vi "Get All CD Parameters.vi"(8 "error in (no error)":errorcluster, 11 "Device Reference in":T17 format="%.0x") -> (0 "error out":errorcluster, 2 "VS References":T1={"Properties"={"Name"="", "CAN"={"Database File"=path "", "CAN Interface"=enum."CAN1", "Baud Rate"=0, "Diagnostic Protocol"=enum."GMLAN", "Transport Protocol"=enum."ISO TP - Normal Mode", "Transmit ID"=0, "Receive ID"=0, "Transmit Extension"=2, "Receive Extension"=1, "Receive UUDT ID"=0, "Enable Stream"=TRUE, "VW TP Channel ID"=0, "Security"={"DLL Path"=path "", "Security Level"=0}}, "FPGA Settings"={"RT Bitfile Path"=path "", "RIO Device"=0, "Enable"=FALSE}, "PIDs"=[], "PID Lookup"=variant(enum16{"GMLAN", "KWP-2000", "UDS"} enum."GMLAN"), "CPIDs"=[], "CPID Lookup"=variant(u32 0), "DIDs"=[], "DID Lookup"=variant(u8 0), "DPIDs"=[], "DPID Lookup"=variant(u32 0), "DTC descriptor"={"DTC Byte Length"=2, "Status Byte Length"=1, "Add Data Byte Length"=1, "Byte Order"=enum."Motorola"}}, "Refs"={"PIDs"=[], "CPIDs"={"Refs"=[], "Values"=[]}, "DIDs"=[], "Number of DTCs"=0, "DTCs"=[], "Success"=0, "Command Chanels"=[]}} {"Refs"."Command Chanels" format="%.0x"; "Refs"."Success" format="%.0x"; "Refs"."DTCs" format="%.0x"; "Refs"."Number of DTCs" format="%.0x"; "Refs"."DIDs" format="%.0x"; "Refs"."CPIDs"."Refs"."Data Reference" format="%.0x"; "Refs"."PIDs" format="%.0x"; "Properties"."CPIDs"."Signals"."Byte Order" items=["Little Endian", "Big Endian"]; "Properties"."CPIDs"."Signals"."Data Type" items=["Signed", "Unsigned", "IEEE Float"]; "Properties"."DIDs"."Signals"."Byte Order" items=["Little Endian", "Big Endian"]; "Properties"."DIDs"."Signals"."Data Type" items=["Signed", "Unsigned", "IEEE Float"]; "Properties"."CAN"."VW TP Channel ID" format="%.0x"; "Properties"."CAN"."Receive UUDT ID" format="%.0x"; "Properties"."CAN"."Receive Extension" format="%.0x"; "Properties"."CAN"."Transmit Extension" format="%.0x"; "Properties"."CAN"."Receive ID" format="%.0x"; "Properties"."CAN"."Transmit ID" format="%.0x"; "Properties"."PIDs"."Signals"."Byte Order" items=["Little Endian", "Big Endian"]; "Properties"."PIDs"."Signals"."Data Type" items=["Signed", "Unsigned", "IEEE Float"]}, 3 "Device Reference out":T17 format="%.0x")   [LabVIEW 2015, in "Diagnostics Addon System Explorer.lvlib"]
uses:
  System Explorer/Diagnostics Addon System Explorer.lvlib
  <vilib>/NI Veristand/Custom Device API/Custom Device Item Ref.ctl
  Compiled.Settings
  Section Properties.ctl
  Shared/CAN Configuration.ctl
  Shared/CAN Interface.ctl
  Shared/Diagnostic Protocols.ctl
  Shared/Transport Protocols.ctl
  Shared/Security.ctl
  Shared/FPGA Bitfile Settings.ctl
  Shared/Frame Parameters.ctl
  Shared/Signal Parameters.ctl
  Shared/DPID Parameters.ctl
  Shared/DPID Periodic Rate.ctl
  <vilib>/Automotive Diagnostic Command Set/Diagnostic Protocols.llb/DTC Descriptor.ctl
  Shared/Compiled.Refs.ctl
  <vilib>/NI Veristand/Custom Device API/Data Reference.ctl
  <vilib>/NI Veristand/Custom Device API/Block Data Reference.ctl
  <vilib>/NI Veristand/Custom Device API/Data Access Type.ctl
  Shared/FG Action.ctl
  Shared/ID FG.vi
  Shared/Get Frame.vi
  System Explorer/SubVIs/Calculate Frame Size.vi
  Shared/Get Signals.vi
  Shared/Signal Parameters FG.vi
  <vilib>/NI Veristand/Custom Device API/NI VeriStand - Get Item Property.vi
  <vilib>/NI Veristand/Custom Device API/Get Item Property (U32 Array).vi
  <vilib>/NI Veristand/Custom Device API/Get Item Property (U32).vi
  <vilib>/NI Veristand/Custom Device API/NI VeriStand - Set Item Property.vi
  <vilib>/NI Veristand/Custom Device API/Set Item Property (U32).vi
  Shared/GUID Lookup.vi
  <vilib>/NI Veristand/Custom Device API/Set Item Property (U32 Array).vi
  <vilib>/NI Veristand/Custom Device Tools/Custom Device Utility Library/NI VeriStand - Search for Item by GUID.vi
  <vilib>/NI Veristand/Custom Device API/Set Item Property (Path).vi
  <vilib>/NI Veristand/Custom Device API/Set Item Property (Boolean).vi
  <vilib>/NI Veristand/Custom Device API/Get Item Property (Path).vi
  <vilib>/NI Veristand/Custom Device API/Get Item Property (Boolean).vi
  <vilib>/NI Veristand/Custom Device Tools/Custom Device Utility Library/NI VeriStand - Search for Item by Name.vi
  <vilib>/NI Veristand/Custom Device API/Get Item Property (I32).vi
  <vilib>/NI Veristand/Custom Device API/Set Item Property (I32).vi
  <vilib>/NI Veristand/Custom Device API/NI VeriStand - Get Custom Device Channel Data.vi
  <vilib>/NI Veristand/Custom Device API/NI VeriStand - Get Item Description.vi
  <vilib>/NI Veristand/Custom Device API/Get Item Property (String).vi
  <vilib>/NI Veristand/Custom Device API/Get Item Property (Double).vi
  <vilib>/NI Veristand/Custom Device API/Set Item Property (String).vi
  <vilib>/NI Veristand/Custom Device API/Set Item Property (Double).vi
  <vilib>/NI Veristand/Custom Device API/NI VeriStand - Get Channel Block Data References.vi
  <vilib>/NI Veristand/Custom Device Tools/Custom Device Utility Library/Custom Device Utility Library.lvlib
  Shared/Diagnostics Addon Shared.lvlib
  <vilib>/NI Veristand/Custom Device API/Custom Device API.lvlib
  Diagnostics Addon Engine.lvlib
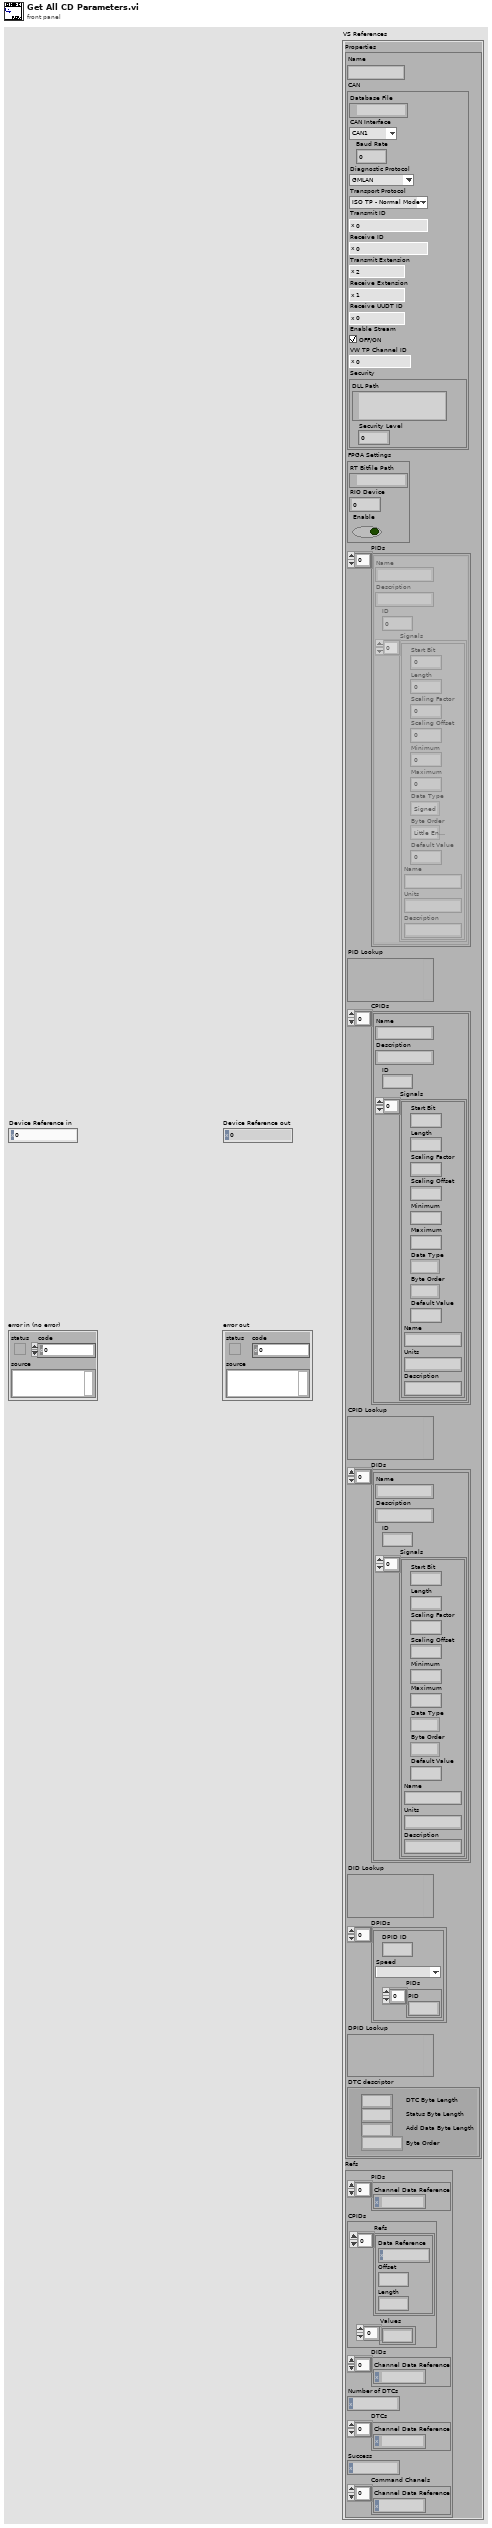
[diagram p1: front panel]
types:
  T1 = typedef "Diagnostics Addon Shared.lvlib/Compiled.Settings" = cluster{"Properties":T2, "Refs":T14}
  T2 = typedef "Diagnostics Addon Engine.lvlib/Section Properties.ctl" = cluster{"Name":string, "CAN":T3, "FPGA Settings":T8, "PIDs":T9[], "PID Lookup":variant, "CPIDs":T9[], "CPID Lookup":variant, "DIDs":T9[], "DID Lookup":variant, "DPIDs":T11[], "DPID Lookup":variant, "DTC descriptor":T13}
  T3 = typedef "Diagnostics Addon Shared.lvlib/CAN Configuration.ctl" = cluster{"Database File":path, "CAN Interface":T4, "Baud Rate":u32, "Diagnostic Protocol":T5, "Transport Protocol":T6, "Transmit ID":u32, "Receive ID":u32, "Transmit Extension":u8, "Receive Extension":u8, "Receive UUDT ID":u32, "Enable Stream":bool, "VW TP Channel ID":u32, "Security":T7}
  T4 = typedef "Diagnostics Addon Shared.lvlib/CAN Interface.ctl" = enum16{"CAN0", "CAN1", "CAN2", "CAN3", "CAN4", "CAN5", "CAN6", "CAN7", "CAN8", "CAN9", "CAN10", "CAN11", "CAN12", "CAN13", "CAN14", "CAN15", "CAN16", "CAN17", "CAN18", "CAN19", "CAN20", "CAN21", "CAN22", "CAN23", "CAN24", "CAN25", "CAN26", "CAN27", "CAN28", "CAN29", "CAN30", "CAN31", "CAN32", "CAN33", "CAN34", "CAN35", "CAN36", "CAN37", "CAN38", "CAN39", "CAN40", "CAN41", "CAN42", "CAN43", "CAN44", "CAN45", "CAN46", "CAN47", "CAN48", "CAN49", "CAN50", "CAN51", "CAN52", "CAN53", "CAN54", "CAN55", "CAN56", "CAN57", "CAN58", "CAN59", "CAN60", "CAN61", "CAN62", "CAN63", "CAN 256 (Virtual)", "CAN 257 (Virtual)"}
  T5 = typedef "Diagnostics Addon Shared.lvlib/Diagnostic Protocols.ctl" = enum16{"GMLAN", "KWP-2000", "UDS"}
  T6 = typedef "Diagnostics Addon Shared.lvlib/Transport Protocols.ctl" = enum16{"ISO TP - Normal Mode", "ISO TP - Mixed Mode", "VW TP 2.0", "Diagnostics on IP"}
  T7 = typedef "Diagnostics Addon Shared.lvlib/Security.ctl" = cluster{"DLL Path":path, "Security Level":u8}
  T8 = typedef "Diagnostics Addon Shared.lvlib/FPGA Bitfile Settings.ctl" = cluster{"RT Bitfile Path":path, "RIO Device":u16, "Enable":bool}
  T9 = typedef "Diagnostics Addon Shared.lvlib/Frame Parameters.ctl" = cluster{"Name":string, "Description":string, "ID":u16, "Signals":T10[]}
  T10 = typedef "Diagnostics Addon Shared.lvlib/Signal Parameters.ctl" = cluster{"Start Bit":u8, "Length":u8, "Scaling Factor":dbl, "Scaling Offset":dbl, "Minimum":dbl, "Maximum":dbl, "Data Type":u32, "Byte Order":u32, "Default Value":dbl, "Name":string, "Units":string, "Description":string}
  T11 = typedef "Diagnostics Addon Shared.lvlib/DPID Parameters.ctl" = cluster{"DPID ID":u8, "Speed":T12, "PIDs":u16[]}
  T12 = typedef "Diagnostics Addon Shared.lvlib/DPID Periodic Rate.ctl" = enum16{"Slow", "Medium", "Fast"}
  T13 = typedef "Diagnostics Addon Shared.lvlib/DTC Descriptor.ctl" = cluster{"DTC Byte Length":i32, "Status Byte Length":i32, "Add Data Byte Length":i32, "Byte Order":enum16{"Motorola", "Intel"}}
  T14 = typedef "Diagnostics Addon Shared.lvlib/Compiled.Refs.ctl" = cluster{"PIDs":T15[], "CPIDs":cluster{"Refs":T16[], "Values":dbl[]}, "DIDs":T15[], "Number of DTCs":T15, "DTCs":T15[], "Success":T15, "Command Chanels":T15[]}
  T15 = typedef "Custom Device API.lvlib/Data Reference.ctl" = i32
  T16 = typedef "Custom Device API.lvlib/Block Data Reference.ctl" = cluster{"Data Reference":T15, "Offset":u64, "Length":u64}
  T17 = typedef "Custom Device API.lvlib/Custom Device Item Ref.ctl" = u64
  T18 = typedef "Diagnostics Addon System Explorer.lvlib/FG Action.ctl" = enum16{"Get", "Set"}
  T19 = typedef "Custom Device API.lvlib/Data Access Type.ctl" = enum16{"Read", "Write"}
  T20 = typedef "Diagnostics Addon System Explorer.lvlib/Frame Signal VS References.ctl" = cluster{"ID":u16, "Signal Refs":T17[]}
  T21 = typedef "Custom Device API.lvlib/Custom Device Item Info.ctl" = cluster{"Name":string, "Is Channel":bool, "GUID":string, "Is Waveform":bool}
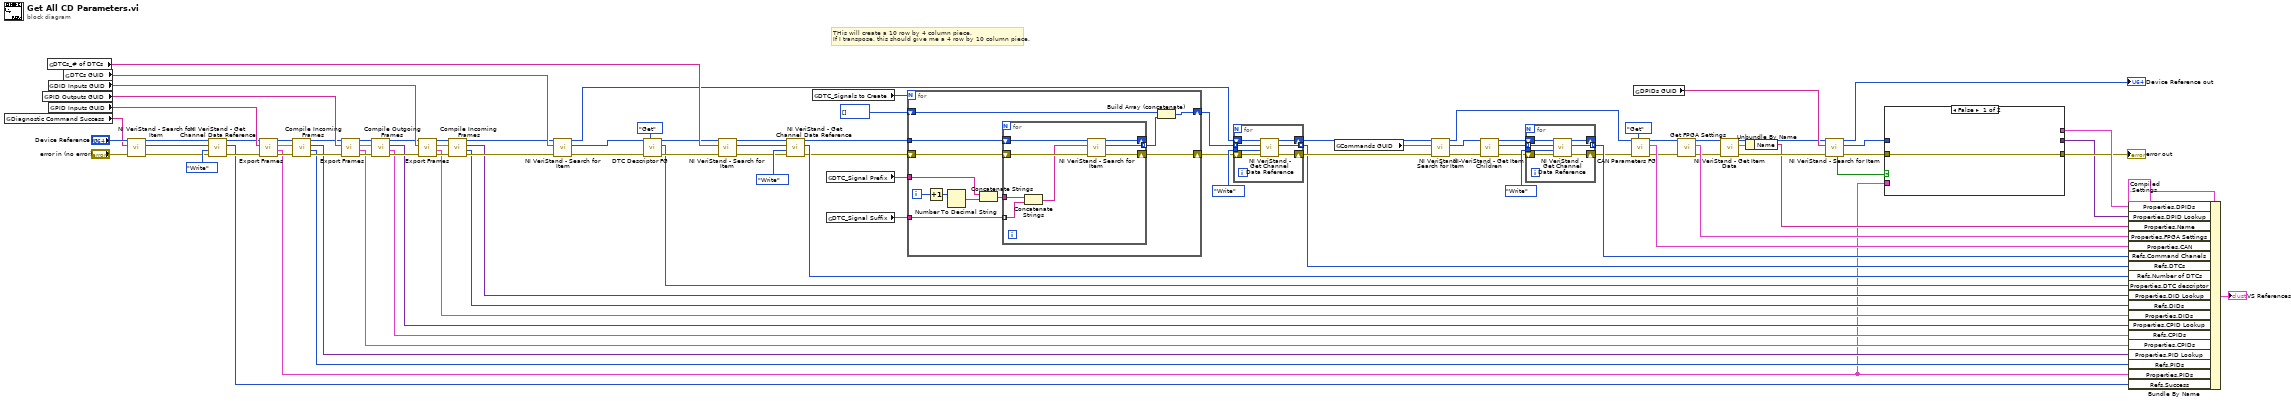
[diagram p0: block diagram]
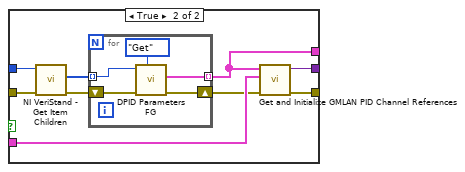
[diagram p2: hidden frame]
diagram:
  # "THis will create a 10 row by 4 column piece.\nIf I transpose, this should give me a 4 row by 10 column piece."
  n1 = global read "GUID Lookup.vi" "Diagnostic Command Success"() -> (w87:string)
  n2 = global read "GUID Lookup.vi" "PID Outputs GUID"() -> (w81:string)
  n3 = global read "GUID Lookup.vi" "DTCs_# of DTCs"() -> (w93:string)
  n4 = global read "GUID Lookup.vi" "DID Inputs GUID"() -> (w82:string)
  n5 = global read "GUID Lookup.vi" "PID Inputs GUID"() -> (w80:string)
  n6 = global read "GUID Lookup.vi" "DTCs GUID"() -> (w94:string)
  n7 = call-poly <vilib>:"NI VeriStand - Search for Item.vi"("error in"="error in (no error)", "Item Name"=w87, "Section Ref in"="Device Reference in") -> ("error out"=w45:errorcluster, "Item Ref"=w41:T17, "Section Ref out"=w43:T17)  [unwired: 5 in, 1 out]
  n8 = call <vilib>:"NI VeriStand - Get Channel Data Reference.vi"("error in (no error)"=w45, "Access"=Data_Access_Type."Write", "Channel Ref in"=w41, "Device Ref in"=w43) -> ("error out"=w44:errorcluster, "Channel Data Reference"=w40:T15, "Device Ref out"=w42:T17)  [unwired: 5 in]
  n9 = call "Export Frames.vi"("error in (no error)"=w44, "GUID"=w80, "Section Ref in"=w42) -> ("error out"=w72:errorcluster, "Frame Settings Array"=w3:T9[], "Frame Refs"=w70:T20[], "Section Ref out"=w74:T17)  [unwired: 5 in]
  n10 = call "Compile Incoming Frames.vi"("error in (no error)"=w72, "Refs"=w70, "Item Ref in"=w74) -> ("error out"=w71:errorcluster, "Refs"=w39:T15[], "Lookup Table"=w23:variant, "Item Ref out"=w73:T17)  [unwired: 5 in]
  n11 = call "Export Frames.vi"("error in (no error)"=w71, "GUID"=w81, "Section Ref in"=w73) -> ("error out"=w64:errorcluster, "Frame Settings Array"=w22:T9[], "Frame Refs"=w60:T20[], "Section Ref out"=w62:T17)  [unwired: 5 in]
  n12 = call "Compile Outgoing Frames.vi"("error in (no error)"=w64, "Refs"=w60, "Item Ref in"=w62) -> ("error out"=w63:errorcluster, "output cluster"=w38:cluster{"Refs":T16[], "Values":dbl[]}, "Lookup Table"=w21:variant, "Item Ref out"=w61:T17)  [unwired: 5 in]
  n13 = call "Export Frames.vi"("error in (no error)"=w63, "GUID"=w82, "Section Ref in"=w61) -> ("error out"=w68:errorcluster, "Frame Settings Array"=w20:T9[], "Frame Refs"=w69:T20[], "Section Ref out"=w66:T17)  [unwired: 5 in]
  n14 = call "Compile Incoming Frames.vi"("error in (no error)"=w68, "Refs"=w69, "Item Ref in"=w66) -> ("error out"=w67:errorcluster, "Refs"=w37:T15[], "Lookup Table"=w19:variant, "Item Ref out"=w65:T17)  [unwired: 5 in]
  n15 = call-poly <vilib>:"NI VeriStand - Search for Item.vi"("error in"=w67, "Item GUID"=w94, "Section Ref in"=w65) -> ("error out"=w28:errorcluster, "Item Ref"=w26:T17, "Section Ref out"=w55:T17)  [unwired: 5 in, 1 out]
  n16 = call "DTC Descriptor FG.vi"("Action"=FG_Action."Get", "error in (no error)"=w28, "Device Item Ref in"=w26) -> ("error out"=w27:errorcluster, "DTC descriptor"=w18:T13, "Device Item Ref out"=w25:T17)  [unwired: 6 in]
  n17 = call-poly <vilib>:"NI VeriStand - Search for Item.vi"("error in"=w27, "Item Name"=w93, "Section Ref in"=w25) -> ("error out"=w50:errorcluster, "Item Ref"=w53:T17, "Section Ref out"=w48:T17)  [unwired: 5 in, 1 out]
  n18 = call <vilib>:"NI VeriStand - Get Channel Data Reference.vi"("error in (no error)"=w50, "Access"=Data_Access_Type."Write", "Channel Ref in"=w53, "Device Ref in"=w48) -> ("error out"=w49:errorcluster, "Channel Data Reference"=w52:T15, "Device Ref out"=w47:T17)  [unwired: 5 in]
  n19 = global read "GUID Lookup.vi" "DTC_Signals to Create"() -> (w90:i32)
  n20 = global read "GUID Lookup.vi" "DTC_Signal Prefix"() -> (w92:string)
  n21 = global read "GUID Lookup.vi" "DTC_Signal Suffix"() -> (w91:string[])
  n22 = for {
    N: w90 -> [_]
    tunnel: w47 -> [w106]
    shift-right: [w104] -> w58
    shift-left: w49 -> [w105]
    tunnel: w91 -> [w99]
    tunnel: w92 -> [w98]
    shift-right: [w95] -> w56
    shift-left: T17[] [] -> [w97]
    i -> [w101]
    n23 = Increment(x=w101) -> (x+1=w103:i32)
    n24 = Number To Decimal String(number=w103) -> (decimal integer string=w102:string)  [unwired: 1 in]
    n25 = Concatenate Strings(w98, w102) -> (w100:string)
    n26 = for {
      shift-right: [w113] -> _
      shift-left: w106 -> [w114]
      shift-right: [w111] -> w104
      shift-left: w105 -> [w112]
      tunnel: w99 -> [w110] mode=indexing
      tunnel: w100 -> [w109]
      tunnel: [w107] -> w96 mode=indexing
      n27 = Concatenate Strings(w109, w110) -> (w108:string)
      n28 = call-poly <vilib>:"NI VeriStand - Search for Item.vi"("error in"=w112, "Item Name"=w108, "Section Ref in"=w114) -> ("error out"=w111:errorcluster, "Item Ref"=w107:T17, "Section Ref out"=w113:T17)  [unwired: 5 in, 1 out]
    }
    n29 = Build Array (concatenate)(w97, w96) -> (w95:T17[])
  }
  n30 = for {
    tunnel: w56 -> [w117] mode=indexing
    tunnel: Data_Access_Type."Write" ("Access") -> [w116]
    shift-right: [w119] -> w57
    shift-left: w58 -> [w120]
    shift-right: [w121] -> w54
    shift-left: w55 -> [w118]
    tunnel: [w115] -> w12 mode=indexing
    n31 = call <vilib>:"NI VeriStand - Get Channel Data Reference.vi"("error in (no error)"=w120, "Access"=w116, "Channel Ref in"=w117, "Device Ref in"=w118) -> ("error out"=w119:errorcluster, "Channel Data Reference"=w115:T15, "Device Ref out"=w121:T17)  [unwired: 5 in]
  }
  n32 = global read "GUID Lookup.vi" "Commands GUID"() -> (w85:string)
  n33 = call-poly <vilib>:"NI VeriStand - Search for Item.vi"("error in"=w57, "Item GUID"=w85, "Section Ref in"=w54) -> ("error out"=w84:errorcluster, "Item Ref"=w83:T17, "Section Ref out"=w30:T17)  [unwired: 5 in, 1 out]
  n34 = call <vilib>:"NI VeriStand - Get Item Children.vi"("error in (no error)"=w84, "Item Ref in"=w83) -> ("error out"=w78:errorcluster, "Child Refs"=w76:T17[], "Item Ref out"=w77:T17)  [unwired: 6 in, 1 out]
  n35 = for {
    tunnel: w76 -> [w124] mode=indexing
    tunnel: Data_Access_Type."Write" ("Access") -> [w123]
    shift-right: [w126] -> w31
    shift-left: w78 -> [w127]
    shift-right: [w128] -> _
    shift-left: w77 -> [w125]
    tunnel: [w122] -> w75 mode=indexing
    n36 = call <vilib>:"NI VeriStand - Get Channel Data Reference.vi"("error in (no error)"=w127, "Access"=w123, "Channel Ref in"=w124, "Device Ref in"=w125) -> ("error out"=w126:errorcluster, "Channel Data Reference"=w122:T15, "Device Ref out"=w128:T17)  [unwired: 5 in]
  }
  n37 = call "CAN Parameters FG.vi"("Action"=FG_Action."Get", "error in (no error)"=w31, "Device Item Ref in"=w30) -> ("error out"=w15:errorcluster, "Diagnostics Basic Configuraiton"=w16:T3, "Device Item Ref out"=w14:T17)  [unwired: 6 in]
  n38 = global read "GUID Lookup.vi" "DPIDs GUID"() -> (w35:string)
  n39 = call "Get FPGA Settings.vi"("error in (no error)"=w15, "Item Ref in"=w14) -> ("error out"=w8:errorcluster, "FPGA Bitfile Settings"=w13:T8, "Item Ref out"=w6:T17)  [unwired: 7 in]
  n40 = call <vilib>:"NI VeriStand - Get Item Data.vi"("error in (no error)"=w8, "Item Ref in"=w6) -> ("error out"=w7:errorcluster, "Item Info"=w9:T21, "Item Ref out"=w5:T17)  [unwired: 6 in, 1 out]
  n41 = Unbundle By Name(w9) -> ("Name"=w4:string)
  n42 = call-poly <vilib>:"NI VeriStand - Search for Item.vi"("error in"=w7, "Item GUID"=w35, "Section Ref in"=w5) -> ("error out"=w36:errorcluster, "Item Ref"=w34:T17, "Section Ref out"=→"Device Reference out":T17, "Found"=w32:bool)  [unwired: 5 in]
  n43 = case shown="False" w32 {
    tunnel: w36 -> [w129 w138]
    tunnel: w34 -> [_ w135]
    tunnel: [w129 w132] -> w2
    tunnel: [_ w130] -> w17
    tunnel: w3 -> [_ w134]
    tunnel: [_ w131] -> w1
    frame False {
    }
    frame True {
      n44 = call <vilib>:"NI VeriStand - Get Item Children.vi"("error in (no error)"=w138, "Item Ref in"=w135) -> ("error out"=w137:errorcluster, "Child Refs"=w136:T17[])  [unwired: 6 in, 2 out]
      n45 = for {
        tunnel: w136 -> [w142] mode=indexing
        tunnel: [w141] -> w130 mode=indexing
        shift-right: [w140] -> w133
        shift-left: w137 -> [w143]
        n46 = call "DPID Parameters FG.vi"("Action"=FG_Action."Get", "error in (no error)"=w143, "Device Item Ref in"=w142) -> ("error out"=w140:errorcluster, "DPID"=w141:T11)  [unwired: 6 in, 1 out]
      }
      n47 = call "Get and Initialize GMLAN PID Channel References.vi"("error in (no error)"=w133, "PIDs"=w134, "DPIDs"=w130) -> ("error out"=w132:errorcluster, "Lookup Table"=w131:variant)  [unwired: 7 in]
    }
  }
  "error out" <- w2
  n48 = Bundle By Name(cluster=T1 {"Properties"={"Name"="", "CAN"={"Database File"=path "", "CAN Interface"=enum."CAN1", "Baud Rate"=0, "Diagnostic Protocol"=enum."GMLAN", "Transport Protocol"=enum."ISO TP - Normal Mode", "Transmit ID"=0, "Receive ID"=0, "Transmit Extension"=2, "Receive Extension"=1, "Receive UUDT ID"=0, "Enable Stream"=TRUE, "VW TP Channel ID"=0, "Security"={"DLL Path"=path "", "Security Level"=0}}, "FPGA Settings"={"RT Bitfile Path"=path "", "RIO Device"=0, "Enable"=FALSE}, "PIDs"=[], "PID Lookup"=variant(enum16{"GMLAN", "KWP-2000", "UDS"} enum."GMLAN"), "CPIDs"=[], "CPID Lookup"=variant(u32 0), "DIDs"=[], "DID Lookup"=variant(u8 0), "DPIDs"=[], "DPID Lookup"=variant(u32 0), "DTC descriptor"={"DTC Byte Length"=2, "Status Byte Length"=1, "Add Data Byte Length"=1, "Byte Order"=enum."Motorola"}}, "Refs"={"PIDs"=[], "CPIDs"={"Refs"=[], "Values"=[]}, "DIDs"=[], "Number of DTCs"=0, "DTCs"=[], "Success"=0, "Command Chanels"=[]}} ("VS References"), "Properties.DPIDs"=w17, "Properties.DPID Lookup"=w1, "Properties.Name"=w4, "Properties.FPGA Settings"=w13, "Properties.CAN"=w16, "Refs.Command Chanels"=w75, "Refs.DTCs"=w12, "Refs.Number of DTCs"=w52, "Properties.DTC descriptor"=w18, "Properties.DID Lookup"=w19, "Refs.DIDs"=w37, "Properties.DIDs"=w20, "Properties.CPID Lookup"=w21, "Refs.CPIDs"=w38, "Properties.CPIDs"=w22, "Properties.PID Lookup"=w23, "Refs.PIDs"=w39, "Properties.PIDs"=w3, "Refs.Success"=w40) -> (→"VS References":T1)
